vi "Resize CaseStructure By Making Space.vi"(8 "error in (no error)":errorcluster, 10 "Bounds":T1, 11 "CSM-Helper in":refnum<class "CSM-Helper.lvclass">) -> (0 "error out":errorcluster, 1 "DiffBound":T1, 2 "MakeSpace.Rect":T2, 3 "CSM-Helper out":refnum<class "CSM-Helper.lvclass">)   [LabVIEW 2017, in "CSM-Helper.lvclass"]
doc: "### Resize CaseStructure By Making Space.vi\n\n-- <b>Controls</b> --\n- <b>Bounds</b>:\n- <b>CSM-Helper in</b>: CSMHelper input\n\n-- <b>Indicators</b> --\n- <b>DiffBound</b>:\n- <b>MakeSpace.Rect</b>:\n- <b>CSM-Helper out</b>: CSMHelper output"
uses:
  CSM-Helper.lvclass
  <vilib>/Utility/miscctls.llb/LVBoundsTypeDef.ctl
  <vilib>/Utility/miscctls.llb/LVRectTypeDef.ctl
  CSM-Helper.lvclass/CSM-Helper.ctl
  Properties/Read Back Tunnels Refs.vi
  Properties/Read Case Structure Ref.vi
  Properties/Read Block Diagram Ref.vi
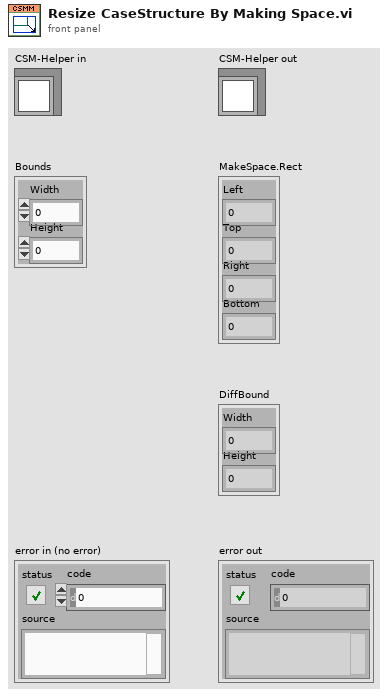
[diagram p1: front panel]
types:
  T1 = typedef "LVBoundsTypeDef.ctl" = cluster{"Width":u32, "Height":u32}
  T2 = typedef "LVRectTypeDef.ctl" = cluster{"Left":i16, "Top":i16, "Right":i16, "Bottom":i16}
  T3 = typedef "CSM-Helper.lvclass/_csmhelper_Back_Tunnels_Refs.ctl" = cluster{"Registration":refnum<vi>, "InternalData":refnum<vi>, "Resp":refnum<vi>, "Remaining State":refnum<vi>, "Error":refnum<vi>}
  T4 = typedef "LVPositionTypeDef.ctl" = cluster{"Left":i32, "Top":i32}
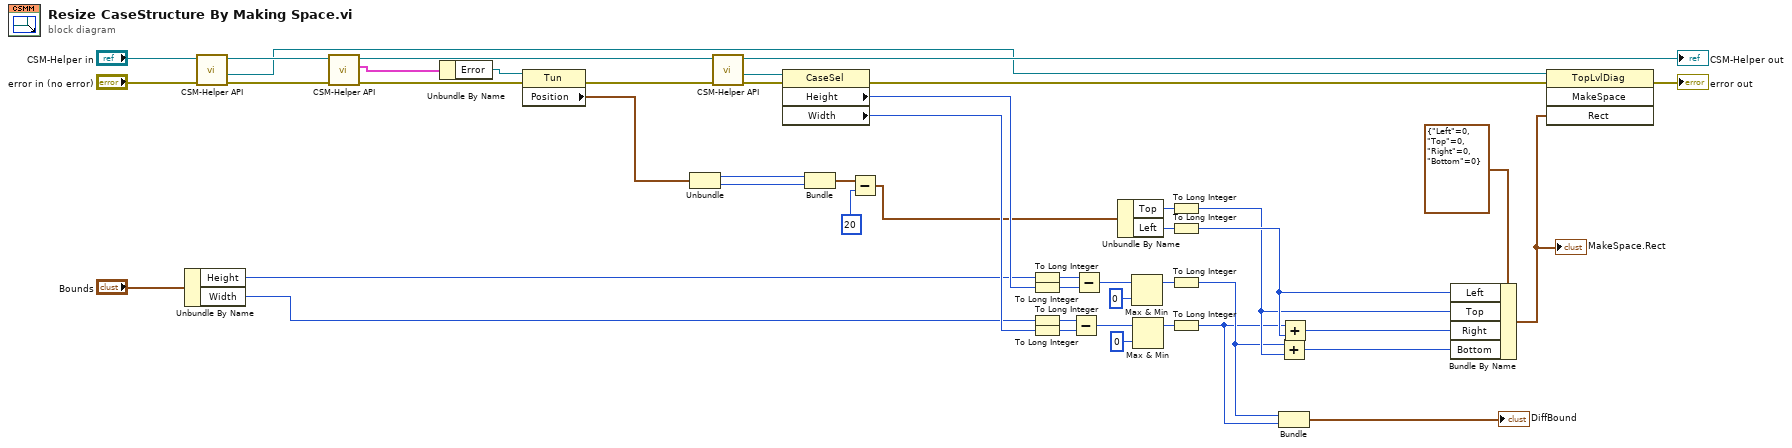
[diagram p0: block diagram]
diagram:
  n1 = Unbundle By Name("Bounds") -> ("Height"=w29:u32, "Width"=w30:u32)
  n2 = call-poly "CSM-Helper API.vi"("error in (no error)"="error in (no error)", "CSM-Helper in"="CSM-Helper in") -> ("error out"=w23:errorcluster, "Diagram"=w14:refnum<vi>, "CSM-Helper out"=w22:refnum<class "CSM-Helper.lvclass">)  [unwired: 7 in]
  n3 = call-poly "CSM-Helper API.vi"("error in (no error)"=w23, "CSM-Helper in"=w22) -> ("error out"=w21:errorcluster, "Back Tunnels"=w18:T3, "CSM-Helper out"=w20:refnum<class "CSM-Helper.lvclass">)  [unwired: 7 in]
  n4 = Unbundle By Name(w18) -> ("Error"=w17:refnum<vi>)
  n5 = property class="Tun"(reference=w17, error in=w21) -> (error out=w19:errorcluster, "Position"=w12:T4)  [unwired: 1 out]
  n6 = Unbundle(w12) -> ("Left"=w11:i32, "Top"=w10:i32)
  n7 = call-poly "CSM-Helper API.vi"("error in (no error)"=w19, "CSM-Helper in"=w20) -> ("error out"=w41:errorcluster, "Case Structure"=w13:refnum<vi>, "CSM-Helper out"=→"CSM-Helper out":refnum<class "CSM-Helper.lvclass">)  [unwired: 7 in]
  n8 = property on="Property Node" class="CaseSel"(reference=w13, error in=w41) -> (error out=w40:errorcluster, "Height"=w39:u32, "Width"=w38:u32)  [unwired: 1 out]
  n9 = Bundle("Left"=w11, "Top"=w10) -> (w9:cluster{"Left":i32, "Top":i32})  [unwired: 1 in]
  n10 = Subtract(x=w9, y=20 ("Height")) -> (x-y=w15:cluster{"Left":i32, "Top":i32})
  n11 = To Long Integer(number=w29) -> (32bit integer=w8:i32)
  n12 = To Long Integer(number=w39) -> (32bit integer=w7:i32)
  n13 = To Long Integer(number=w30) -> (32bit integer=w6:i32)
  n14 = To Long Integer(number=w38) -> (32bit integer=w5:i32)
  n15 = Subtract(x=w6, y=w5) -> (x-y=w36:i32)
  n16 = Subtract(x=w8, y=w7) -> (x-y=w33:i32)
  n17 = Unbundle By Name(w15) -> ("Top"=w28:i32, "Left"=w27:i32)
  n18 = Max & Min(x=w33, y=0) -> (max(x,y)=w25:i32)  [unwired: 1 out]
  n19 = Max & Min(x=w36, y=0) -> (max(x,y)=w26:i32)  [unwired: 1 out]
  n20 = To Long Integer(number=w28) -> (32bit integer=w3:i32)
  n21 = To Long Integer(number=w27) -> (32bit integer=w4:i32)
  n22 = To Long Integer(number=w25) -> (32bit integer=w2:i32)
  n23 = To Long Integer(number=w26) -> (32bit integer=w1:i32)
  n24 = Add(x=w2, y=w3) -> (x+y=w42:i32)
  n25 = Bundle(w2, w1) -> (→"DiffBound":cluster{i32, i32})  [unwired: 1 in]
  n26 = Add(x=w1, y=w4) -> (x+y=w43:i32)
  n27 = Bundle By Name(cluster=T2 {"Left"=0, "Top"=0, "Right"=0, "Bottom"=0} ("Rect"), "Left"=w4, "Top"=w3, "Right"=w43, "Bottom"=w42) -> (w37:T2)
  "MakeSpace.Rect" <- w37
  n28 = invoke on="Invoke Node" class="TopLvlDiag" method="MakeSpace"(reference=w14, error in=w40, "Rect"=w37) -> (error out=→"error out":errorcluster)  [unwired: 1 in, 3 out]
